vi "YKMW100 PRAT Check.vi"() -> ()   [LabVIEW 2019]
uses:
  Trunk/Hybrid Water Heater/Type Definitions/HEWH Power Data.ctl
panel:
  out "Data (Label, Channel, Data) 4":string[][](array[string])
  out "PowerData 4":T1
  out "Data (Label, Channel, Data) 3":string[][](array[string])
  out "PowerData 3":T1
  out "Data (Label, Channel, Data) 2":string[][](array[string])
  out "PowerData 2":T1
  out "PowerData":T1
  out "Data (Label, Channel, Data)":string[][](array[string])
  in  "millisecond multiple":u32=1000
  in  "stop":bool
  in  "MW100 VISA In":refnum<visa-resource-name>="MW100"
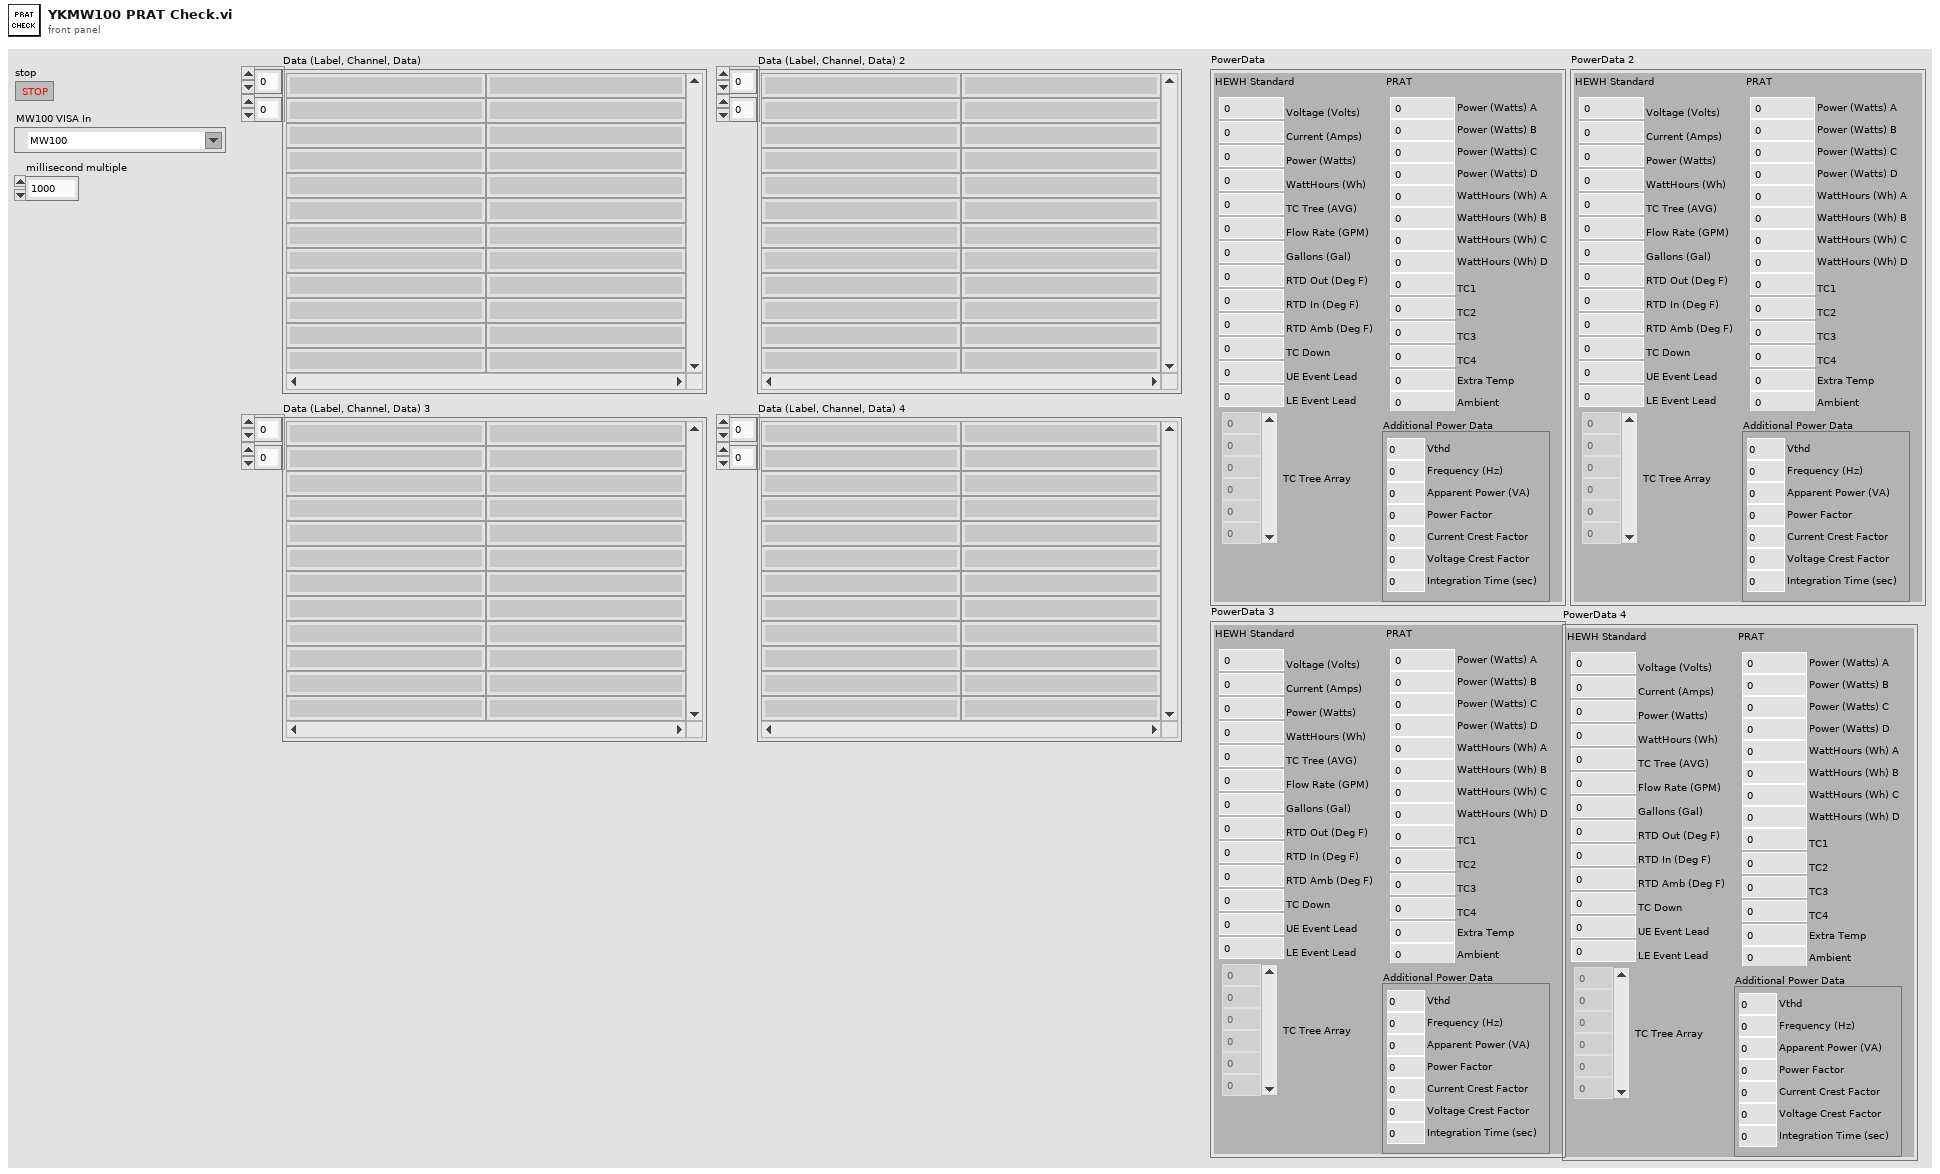
[diagram p1: front panel]
types:
  T1 = typedef "HEWH Power Data.ctl" = cluster{"HEWH Standard":cluster{"Voltage (Volts)":dbl, "Current (Amps)":dbl, "Power (Watts)":dbl, "WattHours (Wh)":dbl, "TC Tree (AVG)":dbl, "Flow Rate (GPM)":dbl, "Gallons (Gal)":dbl, "RTD Out (Deg F)":dbl, "RTD In (Deg F)":dbl, "RTD Amb (Deg F)":dbl, "TC Down":dbl, "UE Event Lead":i32, "LE Event Lead":i32, "TC Tree Array":dbl[]}, "PRAT":cluster{"Power (Watts) A":dbl, "Power (Watts) B":dbl, "Power (Watts) C":dbl, "Power (Watts) D":dbl, "TC1":dbl, "TC2":dbl, "TC3":dbl, "TC4":dbl, "WattHours (Wh) A":dbl, "WattHours (Wh) B":dbl, "WattHours (Wh) C":dbl, "WattHours (Wh) D":dbl, "Ambient":dbl, "Extra Temp":dbl}, "Additional Power Data":cluster{"Vthd":dbl, "Frequency (Hz)":dbl, "Apparent Power (VA)":dbl, "Power Factor":dbl, "Current Crest Factor":dbl, "Voltage Crest Factor":dbl, "Integration Time (sec)":dbl}}
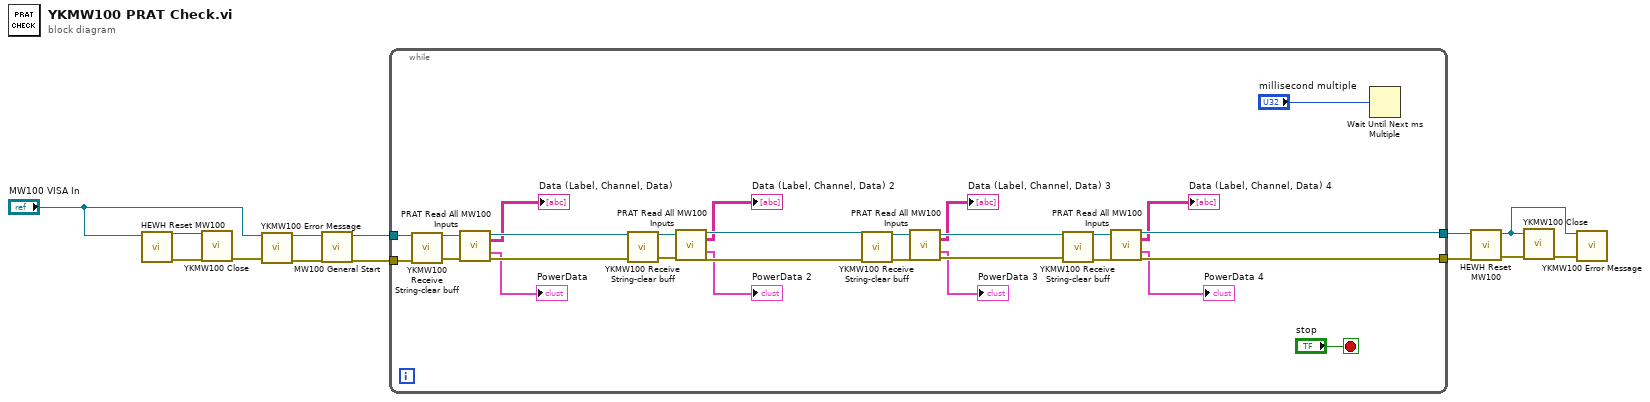
[diagram p0: block diagram]
diagram:
  n1 = call "HEWH Reset MW100.vi"("MW100 VISA In"="MW100 VISA In") -> ("error out"=w11:errorcluster, "MW100 VISA Out"=w13:refnum<visa-resource-name>)  [unwired: 9 in]
  n2 = call "YKMW100 Close.vi"("VISA session"=w13, "error in (no error)"=w11) -> ("error out"=w10:errorcluster)  [unwired: 13 in]
  n3 = call "YKMW100 Error Message.vi"("VISA session"="MW100 VISA In", "error in (no error)"=w10) -> ("dup VISA session"=w3:refnum<visa-resource-name>, "error out"=w4:errorcluster)  [unwired: 9 in, 3 out]
  n4 = call "MW100 General Start.vi"("error in (no error)"=w4, "MW100 Input"=w3) -> ("error out"=w1:errorcluster, "MW100 Output"=w2:refnum<visa-resource-name>)  [unwired: 8 in]
  n5 = while {
    tunnel: [w25] -> w8
    tunnel: [w24] -> w9
    tunnel: w2 -> [w37]
    tunnel: w1 -> [w36]
    stop <- "stop" stop-if-true
    n6 = call "YKMW100 Receive String-clear buff.vi"("VISA session"=w37, "error in (no error)"=w36) -> ("dup VISA session"=w40:refnum<visa-resource-name>, "error out"=w41:errorcluster)  [unwired: 11 in, 1 out]
    n7 = call "PRAT Read All MW100 Inputs.vi"("MW100"=w40, "Error In"=w41) -> ("dup VISA session"=w30:refnum<visa-resource-name>, "Data (Label, Channel, Data)"=→"Data (Label, Channel, Data)":string[][], "PowerData"=→"PowerData":T1, "error out"=w31:errorcluster)  [unwired: 10 in]
    n8 = call "YKMW100 Receive String-clear buff.vi"("VISA session"=w30, "error in (no error)"=w31) -> ("dup VISA session"=w35:refnum<visa-resource-name>, "error out"=w34:errorcluster)  [unwired: 11 in, 1 out]
    n9 = call "PRAT Read All MW100 Inputs.vi"("MW100"=w35, "Error In"=w34) -> ("dup VISA session"=w29:refnum<visa-resource-name>, "Data (Label, Channel, Data)"=→"Data (Label, Channel, Data) 2":string[][], "PowerData"=→"PowerData 2":T1, "error out"=w28:errorcluster)  [unwired: 10 in]
    n10 = call "YKMW100 Receive String-clear buff.vi"("VISA session"=w29, "error in (no error)"=w28) -> ("dup VISA session"=w33:refnum<visa-resource-name>, "error out"=w15:errorcluster)  [unwired: 11 in, 1 out]
    n11 = call "PRAT Read All MW100 Inputs.vi"("MW100"=w33, "Error In"=w15) -> ("dup VISA session"=w26:refnum<visa-resource-name>, "Data (Label, Channel, Data)"=→"Data (Label, Channel, Data) 3":string[][], "PowerData"=→"PowerData 3":T1, "error out"=w27:errorcluster)  [unwired: 10 in]
    n12 = call "YKMW100 Receive String-clear buff.vi"("VISA session"=w26, "error in (no error)"=w27) -> ("dup VISA session"=w32:refnum<visa-resource-name>, "error out"=w14:errorcluster)  [unwired: 11 in, 1 out]
    n13 = call "PRAT Read All MW100 Inputs.vi"("MW100"=w32, "Error In"=w14) -> ("dup VISA session"=w25:refnum<visa-resource-name>, "Data (Label, Channel, Data)"=→"Data (Label, Channel, Data) 4":string[][], "PowerData"=→"PowerData 4":T1, "error out"=w24:errorcluster)  [unwired: 10 in]
    n14 = Wait Until Next ms Multiple(millisecond multiple="millisecond multiple") -> ()  [unwired: 1 out]
  }
  n15 = call "HEWH Reset MW100.vi"("error in (no error)"=w9, "MW100 VISA In"=w8) -> ("error out"=w7:errorcluster, "MW100 VISA Out"=w6:refnum<visa-resource-name>)  [unwired: 8 in]
  n16 = call "YKMW100 Close.vi"("VISA session"=w6, "error in (no error)"=w7) -> ("error out"=w5:errorcluster)  [unwired: 13 in]
  n17 = call "YKMW100 Error Message.vi"("VISA session"=w6, "error in (no error)"=w5) -> ()  [unwired: 9 in, 5 out]
